vi "InitGlobalVariables.vi"   [LabVIEW 2013]
uses:
  GlobalVariables/CalibrationVolumes.vi
  GlobalVariables/CalibrationState.vi
  GlobalVariables/FittedCurvePolynom.vi
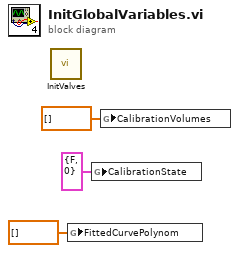
[diagram p0: block diagram]
diagram:
  n1 = call "InitValves.vi"() -> ()  [unwired: 12 in]
  n2 = global write "FittedCurvePolynom.vi" "FittedCurvePolynom"(dbl[] [] ("FittedCurvePolynom")) -> ()
  n3 = global write "CalibrationState.vi" "CalibrationState"(cluster{bool, "CalibrationState":u32} {FALSE, "CalibrationState"=0} ("CalibrationState")) -> ()
  n4 = global write "CalibrationVolumes.vi" "CalibrationVolumes"(dbl[] [] ("CalibrationVolumes")) -> ()
